vi "Stop Core.vi"(10 "final error code":i32, 11 "TCP_Server in":refnum<class "TCP_Server.lvclass">) -> (3 "TCP_Server out":refnum<class "TCP_Server.lvclass">)   [LabVIEW 2023, in "TCP_Server.lvlib" / "TCP_Server.lvclass"]
doc: "(<B>Filename</B>: Actor Framework.lvlib:Actor.lvclass:Stop Core.vi)\n\nDefines what the actor does before it stops. Use the <B>final error code</B> input to determine whether the actor shut down in response to an error.\n\nBy default, this method passes the Stop message along to all auto-stop nested actors. A descendant class may override this method to define additional behavior, such as shutting down any processes the actor initiated in its override of the Actor Core method."
uses:
  TCP_Server.lvclass
  TCP_Server.lvclass/TCP_Server.ctl
  <vilib>/ActorFramework/Message Enqueuer/Message Enqueuer.lvclass/Message Enqueuer.ctl
  <vilib>/ActorFramework/Message Enqueuer/Enqueue.vi
  <vilib>/ActorFramework/Stop Msg/Stop Msg.lvclass
  C:/Program Files (x86)/National Instruments/LabVIEW 2023/vi.lib/ActorFramework/Message/Message.lvclass
  <vilib>/ActorFramework/Message Priority Queue/Priority Enqueue.vi
  <vilib>/ActorFramework/Actor/Actor.lvclass
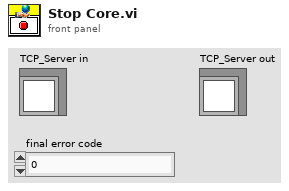
[diagram p1: front panel]
types:
  T1 = typedef "TCP_Server.lvlib/ServerConnection.ctl" = cluster{"Connection Handlers's Enqueuer":refnum<class "Message Enqueuer.lvclass">, "Connection Window's Enqueuer":refnum<class "Message Enqueuer.lvclass">, "Connection Information":T2}
  T2 = typedef "TCP_Listener.lvlib/ConnectionInformation.ctl" = cluster{"Connection number":i32, "Remote Address":string, "Remote Port":u16, "Connection ID":refnum<k5>}
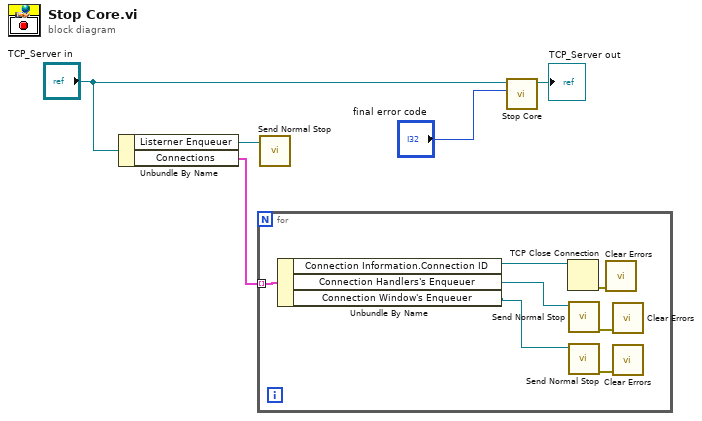
[diagram p0: block diagram]
diagram:
  n1 = Unbundle By Name("TCP_Server in") -> ("Listerner Enqueuer"=w3:refnum<class "Message Enqueuer.lvclass">, "Connections"=w2:T1[])
  n2 = for {
    tunnel: w2 -> [w12] mode=indexing
    n3 = Unbundle By Name(w12) -> ("Connection Information.Connection ID"=w11:refnum<k5>, "Connection Handlers's Enqueuer"=w9:refnum<class "Message Enqueuer.lvclass">, "Connection Window's Enqueuer"=w6:refnum<class "Message Enqueuer.lvclass">)
    n4 = TCP Close Connection(connection ID=w11) -> (error out=w10:errorcluster)  [unwired: 2 in, 1 out]
    n5 = call <vilib>:"Send Normal Stop.vi"("Message Enqueuer"=w9) -> ("error out"=w8:errorcluster)  [unwired: 10 in]
    n6 = call <vilib>:"Send Normal Stop.vi"("Message Enqueuer"=w6) -> ("error out"=w7:errorcluster)  [unwired: 10 in]
    n7 = call <vilib>:"Clear Errors.vi"("error in (no error)"=w10) -> ()  [unwired: 5 in, 2 out]
    n8 = call <vilib>:"Clear Errors.vi"("error in (no error)"=w8) -> ()  [unwired: 5 in, 2 out]
    n9 = call <vilib>:"Clear Errors.vi"("error in (no error)"=w7) -> ()  [unwired: 5 in, 2 out]
  }
  n10 = call <vilib>:"Send Normal Stop.vi"("Message Enqueuer"=w3) -> ()  [unwired: 10 in, 1 out]
  n11 = call-parent "Stop Core.vi"("final error code"="final error code", "Actor in"="TCP_Server in") -> ("Actor out"=→"TCP_Server out":refnum<class "TCP_Server.lvclass">)  [unwired: 9 in]
